vi "PID band check.vi"(7 "DAQ state cluster in":T1 {"T cont"."utility"."therm volt" format="%_6g"; "T cont"."utility"."heat volt in" format="%_6g"; "T cont"."utility"."heat volt out" format="%_6g"; "T cont"."utility"."power out" format="%_6g"; "T cont"."utility"."H Vmax" format="%_6g"; "T cont"."exec"."man power" format="%_6g"; "T cont"."exec"."exec setpoint" format="%_6g"; "T cont"."T params"."Settle Time" step=1.0; "T cont"."T params"."Settle Bandwidth" step=0.01; "T cont"."T params"."Derivative Tme" step=0.01; "T cont"."T params"."Integral Time" step=1.0; "T cont"."T params"."Control Bandwidth" step=0.1; "T cont"."T params"."Setpoint" step=0.1; "T cont"."T status"."Setpoint" format="%_6g"; "T cont"."T status"."Power" format="%_6g"; "T cont"."T status"."Temp" format="%_6g"}) -> (8 "DAQ state cluster out":T1 {"T cont"."utility"."therm volt" format="%_6g"; "T cont"."utility"."heat volt in" format="%_6g"; "T cont"."utility"."heat volt out" format="%_6g"; "T cont"."utility"."power out" format="%_6g"; "T cont"."utility"."H Vmax" format="%_6g"; "T cont"."exec"."man power" format="%_6g"; "T cont"."exec"."exec setpoint" format="%_6g"; "T cont"."T params"."Settle Time" step=1.0; "T cont"."T params"."Settle Bandwidth" step=0.01; "T cont"."T params"."Derivative Tme" step=0.01; "T cont"."T params"."Integral Time" step=1.0; "T cont"."T params"."Control Bandwidth" step=0.1; "T cont"."T params"."Setpoint" step=0.1; "T cont"."T status"."Setpoint" format="%_6g"; "T cont"."T status"."Power" format="%_6g"; "T cont"."T status"."Temp" format="%_6g"}, 12 "In SB":bool, 14 "In CB":bool)   [LabVIEW 2019]
uses:
  typedefs/DAQ T state cluster.ctl
  typedefs/DAQ T state enum.ctl
  typedefs/temp cont cluster.ctl
  typedefs/temp exec cluster.ctl
  typedefs/temp mode enum.ctl
  typedefs/temp indicator.ctl
  typedefs/temp control status.ctl
  typedefs/PID control parameters.ctl
  typedefs/temp cont utility.ctl
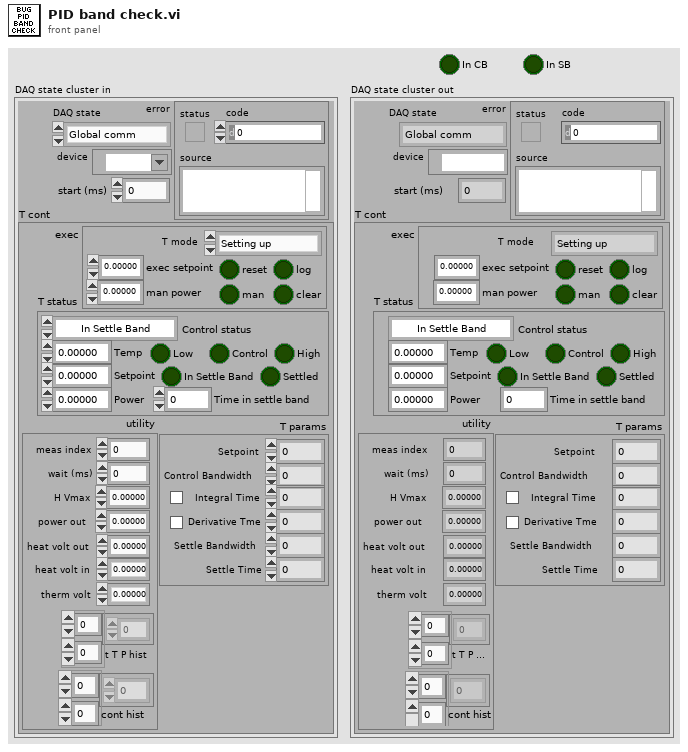
[diagram p1: front panel]
types:
  T1 = typedef "DAQ T state cluster.ctl" = cluster{"DAQ state":T2, "device":tag, "start (ms)":i32, "error":errorcluster, "T cont":T3}
  T2 = typedef "DAQ T state enum.ctl" = enum16{"Global comm", "Meas T & P", "PID power calc", "Man Power set", "Output Power", "Wait", "Exit"}
  T3 = typedef "temp cont cluster.ctl" = cluster{"exec":T4, "T status":T6, "T params":T8, "utility":T9}
  T4 = typedef "temp exec cluster.ctl" = cluster{"T mode":T5, "exec setpoint":dbl, "reset":bool, "man power":dbl, "man":bool, "log":bool, "clear":bool}
  T5 = typedef "temp mode enum.ctl" = enum16{"Setting up", "Listening to exec", "Exit"}
  T6 = typedef "temp indicator.ctl" = cluster{"Control status":T7, "Temp":dbl, "Power":dbl, "Time in settle band":dbl, "Settled":bool, "Low":bool, "High":bool, "Setpoint":dbl, "Control":bool, "In Settle Band":bool}
  T7 = typedef "temp control status.ctl" = enum16{"In Settle Band", "In Control Band", "Below Control Band", "Above Control Band"}
  T8 = typedef "PID control parameters.ctl" = cluster{"Setpoint":dbl, "Control Bandwidth":dbl, "Integral Time":dbl, "Int\nON":bool, "Derivative Tme":dbl, "Der\nON":bool, "Settle Bandwidth":dbl, "Settle Time":dbl}
  T9 = typedef "temp cont utility.ctl" = cluster{"meas index":i32, "wait (ms)":i32, "H Vmax":dbl, "power out":dbl, "heat volt out":dbl, "heat volt in":dbl, "therm volt":dbl, "t T P hist":dbl[][], "cont hist":dbl[][]}
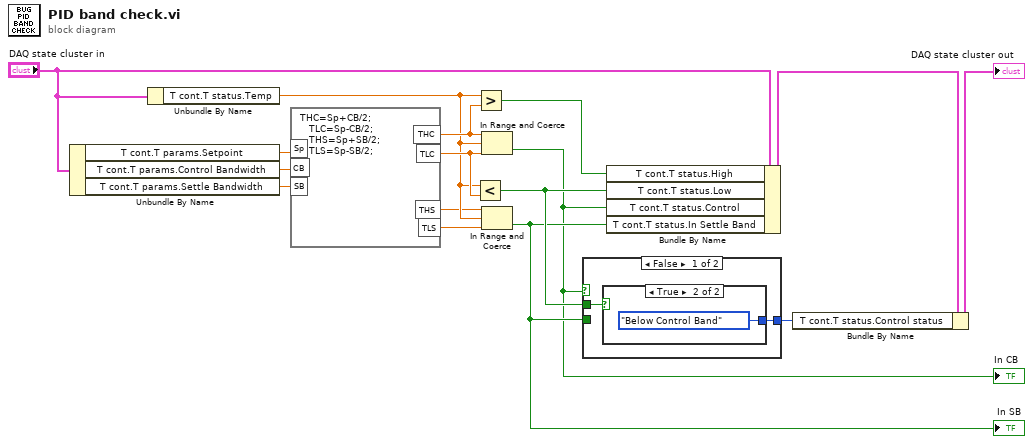
[diagram p0: block diagram]
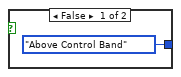
[diagram p2: hidden frame]
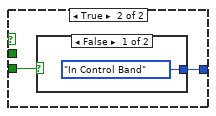
[diagram p3: hidden frame]
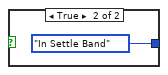
[diagram p4: hidden frame]
diagram:
  n1 = Unbundle By Name("DAQ state cluster in") -> ("T cont.T params.Setpoint"=w7:dbl, "T cont.T params.Control Bandwidth"=w8:dbl, "T cont.T params.Settle Bandwidth"=w9:dbl)
  n2 = Unbundle By Name("DAQ state cluster in") -> ("T cont.T status.Temp"=w12:dbl)
  n3 = formula code="THC=Sp+CB/2;\n   TLC=Sp-CB/2;\n   THS=Sp+SB/2;\n   TLS=Sp-SB/2;"("Sp"=w7, "CB"=w8, "SB"=w9) -> ("THC"=w14:dbl, "TLC"=w15:dbl, "THS"=w11:dbl, "TLS"=w13:dbl)
  n4 = Less?(x=w12, y=w15) -> (x < y?=w3:bool)
  n5 = Greater?(x=w12, y=w14) -> (0:w16:bool)
  n6 = In Range and Coerce(upper limit=w14, x=w12, lower limit=w15) -> (In Range?=w1:bool)  [unwired: 1 out]
  "In CB" <- w1
  n7 = In Range and Coerce(upper limit=w11, x=w12, lower limit=w13) -> (In Range?=w2:bool)  [unwired: 1 out]
  "In SB" <- w2
  n8 = case shown="False" w1 {
    tunnel: [w17 w22] -> w6
    tunnel: w2 -> [_ w21]
    tunnel: w3 -> [w18 _]
    frame False {
      n9 = case shown="True" w18 {
        tunnel: [temp_control_status."Above Control Band" ("T cont.T status.Control status") temp_control_status."Below Control Band" ("T cont.T status.Control status")] -> w17
        frame False {
        }
        frame True {
        }
      }
    }
    frame True {
      n10 = case shown="False" w21 {
        tunnel: [temp_control_status."In Control Band" ("T cont.T status.Control status") temp_control_status."In Settle Band" ("T cont.T status.Control status")] -> w22
        frame False {
        }
        frame True {
        }
      }
    }
  }
  n11 = Bundle By Name(cluster="DAQ state cluster in", "T cont.T status.High"=w16, "T cont.T status.Low"=w3, "T cont.T status.Control"=w1, "T cont.T status.In Settle Band"=w2) -> (w5:T1)
  n12 = Bundle By Name(cluster=w5, "T cont.T status.Control status"=w6) -> (→"DAQ state cluster out":T1)
